vi "main.vi"() -> ()   [LabVIEW 2013]
uses:
  Controls/Soda Drinks.ctl
  Controls/Diet Soda Drinks.ctl
  Controls/Energy Drinks.ctl
  Controls/Alcohol Drinks.ctl
  Controls/Main UI Drinks.ctl
  Controls/Main Enum.ctl
panel:
  in  "cc?":bool
  out "CtlRef":refnum<vi>
  out "Label.Text":string
  in  "stop":bool
  in  "Reference Cluster":T1
  in  "UI":T2(tab)
  in  "All Selections":T3={"DaSani 20oz"=FALSE, "Mt. Dew 12oz"=FALSE, "Mt. Dew 20oz"=FALSE, "Diet Mt. Dew 20oz"=FALSE, "Pepsi 12oz"=FALSE, "Pepsi 20oz"=FALSE, "Diet Pepsi 20oz"=FALSE, "Sprite 12oz"=FALSE, "Sprite 20oz"=FALSE, "Dr. Pepper 12oz"=FALSE, "Dr. Pepper 20oz"=FALSE, "Lipton 16oz"=FALSE, "Starbucks 12oz"=FALSE, "Red Bull 8oz"=FALSE, "Coors 16oz"=FALSE, "Coors Light 16oz"=FALSE, "Hydra 12oz"=FALSE, "Diet Dr. Pepper 20oz"=FALSE, "Mt.Dew 12oz Price"=1.0, "Mt.Dew 20oz Price"=1.5, "Diet Mt.Dew 20oz Price"=1.5, "Pepsi 12oz Price"=1.0, "Pepsi 20oz Price"=1.5, "Diet Pepsi 20oz Price"=1.5, "Sprite 12oz Price"=1.0, "Sprite 20oz Price"=1.5, "Dr. Pepper 12oz Price"=1.0, "Dr. Pepper 20oz Price"=1.5, "Diet Dr. Pepper 20oz Price"=1.5, "DaSani 20oz Price"=1.0, "Lipton Prioce"=1.5, "Starbucks Price"=1.5, "Red Bull Price"=2.0, "Coors Price"=2.0, "Coors Light Price"=2.0, "Hydra Price"=2.0} {"Hydra Price" format="%.2g"; "Coors Light Price" format="%.2g"; "Coors Price" format="%.2g"; "Red Bull Price" format="%.2g"; "Starbucks Price" format="%.2g"; "Lipton Prioce" format="%.2g"; "DaSani 20oz Price" format="%.2g"; "Diet Dr. Pepper 20oz Price" format="%.2g"; "Dr. Pepper 20oz Price" format="%.2g"; "Dr. Pepper 12oz Price" format="%.2g"; "Sprite 20oz Price" format="%.2g"; "Sprite 12oz Price" format="%.2g"; "Diet Pepsi 20oz Price" format="%.2g"; "Pepsi 20oz Price" format="%.2g"; "Pepsi 12oz Price" format="%.2g"; "Diet Mt.Dew 20oz Price" format="%.2g"; "Mt.Dew 20oz Price" format="%.2g"; "Mt.Dew 12oz Price" format="%.2f"}
  in  "Energy":bool
  in  "Diet":bool
  in  "Alcohol":bool
  in  "Soda":bool
  in  "Add Money":bool
  out "Available Funds":dbl format="%.2f"
  in  "Return Money":bool
  out "Available Funds 2":dbl format="%.2f"
  in  "Imploded 1 Cancel":bool
  in  "Soda Drinks":T4={"DaSani 20oz"=FALSE, "Mt. Dew 12oz"=FALSE, "Mt. Dew 20oz"=FALSE, "Diet Mt. Dew 20oz"=FALSE, "Pepsi 12oz"=FALSE, "Pepsi 20oz"=FALSE, "Diet Pepsi 20oz"=FALSE, "Sprite 12oz"=FALSE, "Sprite 20oz"=FALSE, "Dr. Pepper 12oz"=FALSE, "Dr. Pepper 20oz"=FALSE, "Diet Dr. Pepper 20oz"=FALSE, "Mt.Dew 12oz Price"=1.0, "Mt.Dew 20oz Price"=1.5, "Diet Mt.Dew 20oz Price"=1.5, "Pepsi 12oz Price"=1.0, "Pepsi 20oz Price"=1.5, "Diet Pepsi 20oz Price"=1.5, "Sprite 12oz Price"=1.0, "Sprite 20oz Price"=1.5, "Dr. Pepper 12oz Price"=1.0, "Dr. Pepper 20oz Price"=1.5, "Diet Dr. Pepper 20oz Price"=1.5, "DaSani 20oz Price"=1.0} {"DaSani 20oz Price" format="%.2f"; "Diet Dr. Pepper 20oz Price" format="%.2f"; "Dr. Pepper 20oz Price" format="%.2f"; "Dr. Pepper 12oz Price" format="%.2f"; "Sprite 20oz Price" format="%.2f"; "Sprite 12oz Price" format="%.2f"; "Diet Pepsi 20oz Price" format="%.2f"; "Pepsi 20oz Price" format="%.2f"; "Pepsi 12oz Price" format="%.2f"; "Diet Mt.Dew 20oz Price" format="%.2f"; "Mt.Dew 20oz Price" format="%.2f"; "Mt.Dew 12oz Price" format="%.2f"}
  in  "Diet Selections":T5={"DaSani 20oz"=FALSE, "Diet Mt. Dew 20oz"=FALSE, "Diet Pepsi 20oz"=FALSE, "Diet Dr. Pepper 20oz"=FALSE, "Diet Mt.Dew 20oz Price"=1.5, "Diet Pepsi 20oz Price"=1.5, "Diet Dr. Pepper 20oz Price"=1.5, "DaSani 20oz Price"=1.0} {"DaSani 20oz Price" format="%.2f"; "Diet Dr. Pepper 20oz Price" format="%.2f"; "Diet Pepsi 20oz Price" format="%.2f"; "Diet Mt.Dew 20oz Price" format="%.2f"}
  in  "Energy Selections":T6={"Lipton 16oz"=FALSE, "Starbucks 12oz"=FALSE, "Red Bull 8oz"=FALSE, "Lipton Prioce"=1.5, "Starbucks Price"=1.5, "Red Bull Price"=2.0} {"Red Bull Price" format="%.2f"; "Starbucks Price" format="%.2f"; "Lipton Prioce" format="%.2f"}
  in  "Alcohol Drinks":T7={"Coors 16oz"=FALSE, "Coors Light 16oz"=FALSE, "Hydra 12oz"=FALSE, "Coors Price"=2.0, "Coors Light Price"=2.0, "Hydra Price"=2.0} {"Hydra Price" format="%.2f"; "Coors Light Price" format="%.2f"; "Coors Price" format="%.2f"}
  in  "Diet Implode":bool
  in  "Add Money 2":bool
  out "Available Funds 3":dbl format="%.2f"
  in  "Imploded 2 Cancel":bool
  in  "Diet Selections 2":T5={"DaSani 20oz"=FALSE, "Diet Mt. Dew 20oz"=FALSE, "Diet Pepsi 20oz"=FALSE, "Diet Dr. Pepper 20oz"=FALSE, "Diet Mt.Dew 20oz Price"=1.5, "Diet Pepsi 20oz Price"=1.5, "Diet Dr. Pepper 20oz Price"=1.5, "DaSani 20oz Price"=1.0} {"DaSani 20oz Price" format="%.2g"; "Diet Dr. Pepper 20oz Price" format="%.2g"; "Diet Pepsi 20oz Price" format="%.2g"; "Diet Mt.Dew 20oz Price" format="%.2g"}
  in  "Add Money 3":bool
  in  "Credit Card Cancel":bool
  in  "ID Scan Cancel":bool
  in  "Breath Cancel":bool
  in  "EXIT":bool
  # "In the actual implemented User Interface this lower section will not be developed.\nThis program is to only be used as a simulation of the application and how the UI \nshould work in various situations. \nAlso this is nowhere near a final UI it is a super duper rough draft :)\nMerely so I understand better what it is the system will accomplish."
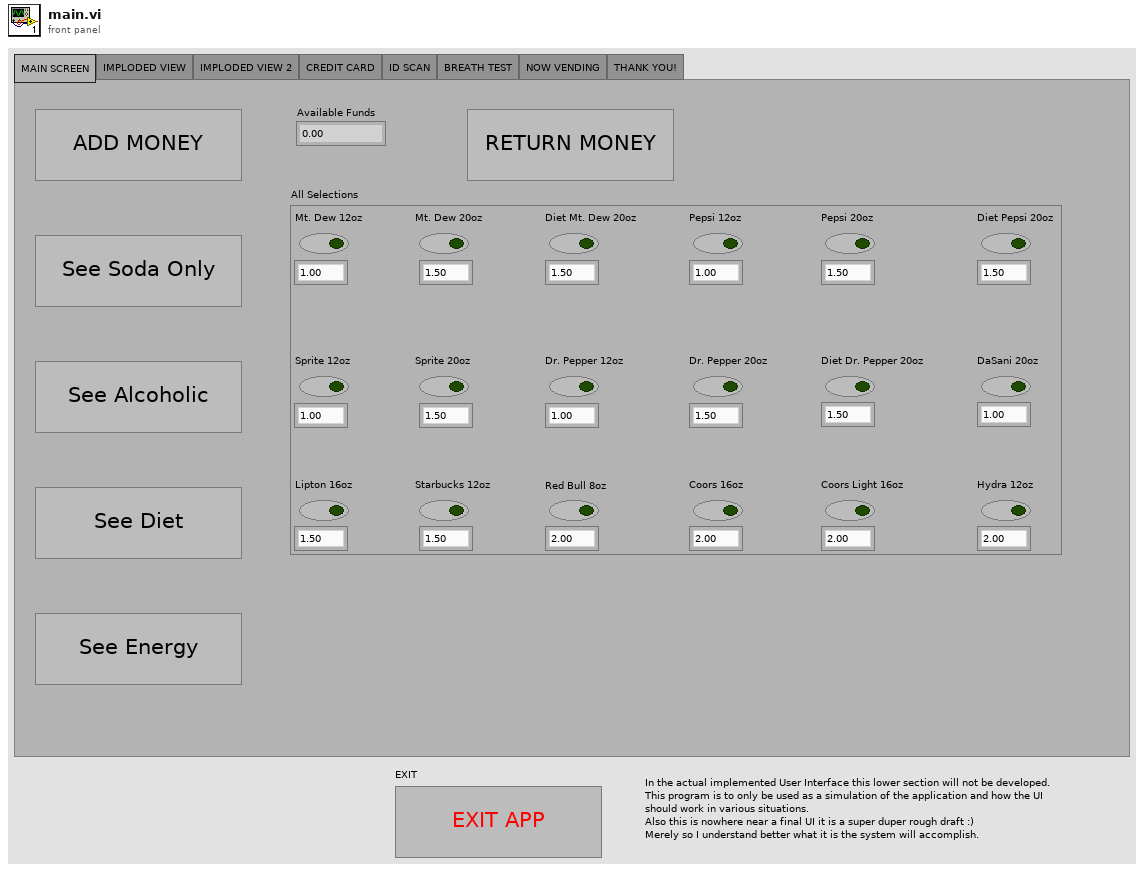
[diagram p1: front panel]
types:
  T1 = cluster{"Alcohol Drinks":refnum<vi>, "Energy Selections":refnum<vi>, "Diet Selections":refnum<vi>, "Soda Drinks":refnum<vi>}
  T2 = enum32{"MAIN SCREEN", "IMPLODED VIEW", "IMPLODED VIEW 2", "CREDIT CARD", "ID SCAN", "BREATH TEST", "NOW VENDING", "THANK YOU!"}
  T3 = typedef "Main UI Drinks.ctl" = cluster{"DaSani 20oz":bool, "Mt. Dew 12oz":bool, "Mt. Dew 20oz":bool, "Diet Mt. Dew 20oz":bool, "Pepsi 12oz":bool, "Pepsi 20oz":bool, "Diet Pepsi 20oz":bool, "Sprite 12oz":bool, "Sprite 20oz":bool, "Dr. Pepper 12oz":bool, "Dr. Pepper 20oz":bool, "Lipton 16oz":bool, "Starbucks 12oz":bool, "Red Bull 8oz":bool, "Coors 16oz":bool, "Coors Light 16oz":bool, "Hydra 12oz":bool, "Diet Dr. Pepper 20oz":bool, "Mt.Dew 12oz Price":dbl, "Mt.Dew 20oz Price":dbl, "Diet Mt.Dew 20oz Price":dbl, "Pepsi 12oz Price":dbl, "Pepsi 20oz Price":dbl, "Diet Pepsi 20oz Price":dbl, "Sprite 12oz Price":dbl, "Sprite 20oz Price":dbl, "Dr. Pepper 12oz Price":dbl, "Dr. Pepper 20oz Price":dbl, "Diet Dr. Pepper 20oz Price":dbl, "DaSani 20oz Price":dbl, "Lipton Prioce":dbl, "Starbucks Price":dbl, "Red Bull Price":dbl, "Coors Price":dbl, "Coors Light Price":dbl, "Hydra Price":dbl}
  T4 = typedef "Soda Drinks.ctl" = cluster{"DaSani 20oz":bool, "Mt. Dew 12oz":bool, "Mt. Dew 20oz":bool, "Diet Mt. Dew 20oz":bool, "Pepsi 12oz":bool, "Pepsi 20oz":bool, "Diet Pepsi 20oz":bool, "Sprite 12oz":bool, "Sprite 20oz":bool, "Dr. Pepper 12oz":bool, "Dr. Pepper 20oz":bool, "Diet Dr. Pepper 20oz":bool, "Mt.Dew 12oz Price":dbl, "Mt.Dew 20oz Price":dbl, "Diet Mt.Dew 20oz Price":dbl, "Pepsi 12oz Price":dbl, "Pepsi 20oz Price":dbl, "Diet Pepsi 20oz Price":dbl, "Sprite 12oz Price":dbl, "Sprite 20oz Price":dbl, "Dr. Pepper 12oz Price":dbl, "Dr. Pepper 20oz Price":dbl, "Diet Dr. Pepper 20oz Price":dbl, "DaSani 20oz Price":dbl}
  T5 = typedef "Diet Soda Drinks.ctl" = cluster{"DaSani 20oz":bool, "Diet Mt. Dew 20oz":bool, "Diet Pepsi 20oz":bool, "Diet Dr. Pepper 20oz":bool, "Diet Mt.Dew 20oz Price":dbl, "Diet Pepsi 20oz Price":dbl, "Diet Dr. Pepper 20oz Price":dbl, "DaSani 20oz Price":dbl}
  T6 = typedef "Energy Drinks.ctl" = cluster{"Lipton 16oz":bool, "Starbucks 12oz":bool, "Red Bull 8oz":bool, "Lipton Prioce":dbl, "Starbucks Price":dbl, "Red Bull Price":dbl}
  T7 = typedef "Alcohol Drinks.ctl" = cluster{"Coors 16oz":bool, "Coors Light 16oz":bool, "Hydra 12oz":bool, "Coors Price":dbl, "Coors Light Price":dbl, "Hydra Price":dbl}
  T8 = typedef "Main Enum.ctl" = enum8{"Initialize", "Timeout", "Add Money", "Return Money", "Implode Soda", "Implode Alcohol", "Implode Diet", "Implode Energy", "Secondary Implode", "Credit Card", "ID Scan", "Breath Test", "Vending", "Thanks!", "Reset to Default", "Exit", "Deinitialize"}
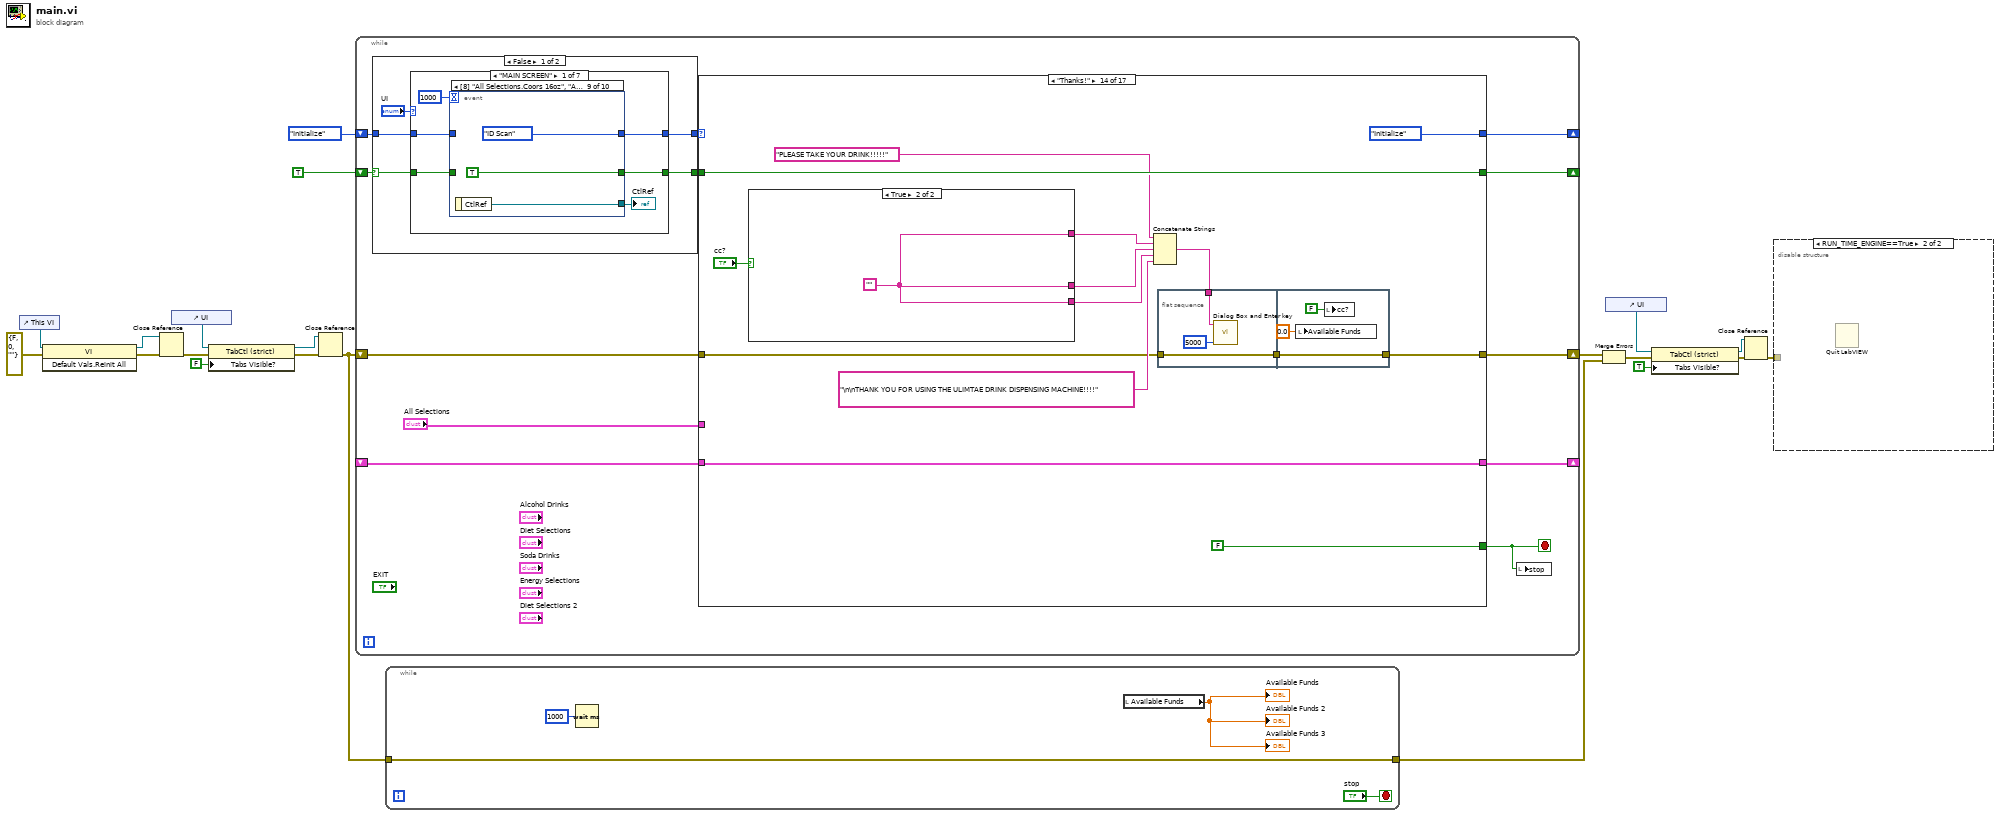
[diagram p0: block diagram]
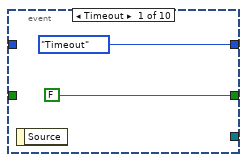
[diagram p3: hidden frame]
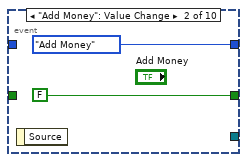
[diagram p4: hidden frame]
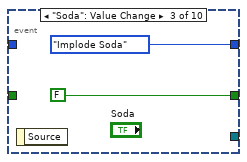
[diagram p5: hidden frame]
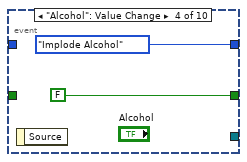
[diagram p6: hidden frame]
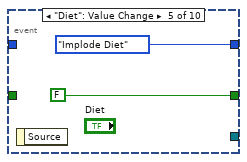
[diagram p7: hidden frame]
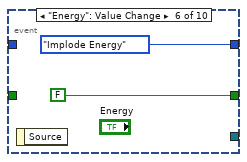
[diagram p8: hidden frame]
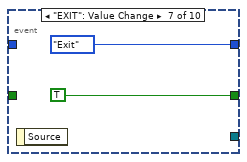
[diagram p9: hidden frame]
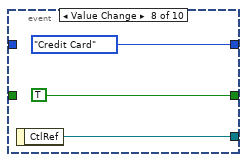
[diagram p10: hidden frame]
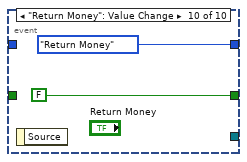
[diagram p11: hidden frame]
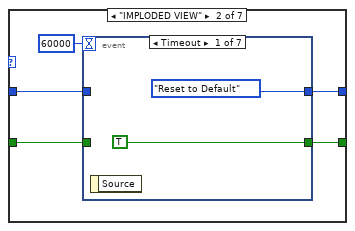
[diagram p12: hidden frame]
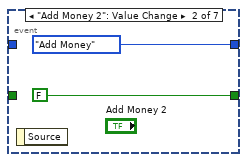
[diagram p13: hidden frame]
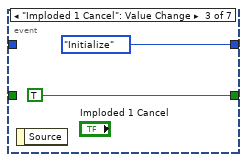
[diagram p14: hidden frame]
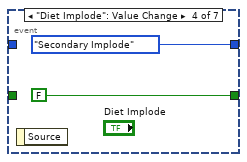
[diagram p15: hidden frame]
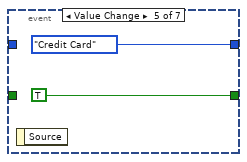
[diagram p16: hidden frame]
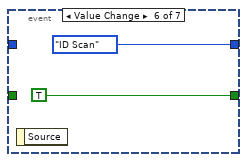
[diagram p17: hidden frame]
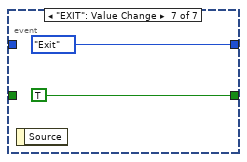
[diagram p18: hidden frame]
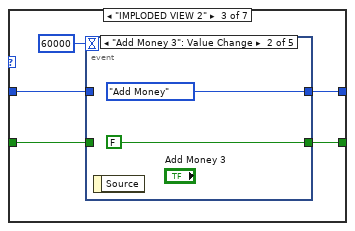
[diagram p19: hidden frame]
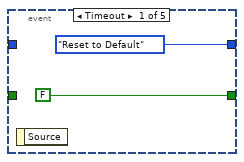
[diagram p20: hidden frame]
diagram:
  n1 = control-ref of="This VI"() -> (w3:refnum<vi>)
  n2 = invoke class="VI" method="Default Vals.Reinit All"(reference=w3, error in=errorcluster {"status"=FALSE, "code"=0, "source"=""} ("error constant")) -> (reference out=w5:refnum<vi>, error out=w4:errorcluster)  [unwired: 1 in, 1 out]
  n3 = Close Reference(reference=w5, error in (no error)=w4) -> (error out=w1:errorcluster)
  n4 = control-ref of="UI"() -> (w18:refnum<vi>)
  n5 = property class="TabCtl (strict)"(reference=w18, error in=w1, "Tabs Visible?"=FALSE) -> (reference out=w15:refnum<vi>, error out=w16:errorcluster)
  n6 = Close Reference(reference=w15, error in (no error)=w16) -> (error out=w7:errorcluster)
  n7 = while {
    shift-right: [w27] -> _
    shift-left: Main_Enum."Initialize" ("Enum") -> [w32]
    shift-right: [w28] -> _
    shift-left: TRUE -> [w31]
    shift-right: [w25] -> w9
    shift-left: w7 -> [w26]
    shift-right: [w22] -> _
    shift-left: _ -> [w23]
    stop <- w24 stop-if-true
    n8 = case shown="False" w31 {
      selector: w31 -> [w36 w135]
      tunnel: w32 -> [w35 w136]
      tunnel: [w34 w136] -> w29
      tunnel: [w33 w135] -> w30
      frame False {
        n9 = case shown="\"MAIN SCREEN\"" "UI" {
          tunnel: w36 -> [w41 w68 w87 w102 w113 w124 w133]
          tunnel: w35 -> [w42 w69 w88 w103 w114 w125 w134]
          tunnel: [w40 w67 w86 w101 w112 w123 w134] -> w34
          tunnel: [w39 w66 w85 w100 w111 w122 w133] -> w33
          frame "MAIN SCREEN" {
            n10 = event shown="[8] \"All Selections.Coors 16oz\", \"All Selections.Coors Light 16oz\", \"All Selections.Hydra 12oz\": Value Change" {
              selector: _ -> [_ _ _ _ _ _ _ _ _ _]
              dyn-events: _ -> [_ _ _ _ _ _ _ _ _ _]
              timeout: 1000 -> [_ _ _ _ _ _ _ _ _ _]
              tunnel: w42 -> [_ _ _ _ _ _ _ _ _ _]
              tunnel: w41 -> [_ _ _ _ _ _ _ _ _ _]
              tunnel: [Main_Enum."Timeout" ("Enum") Main_Enum."Add Money" ("Enum") Main_Enum."Implode Soda" ("Enum") Main_Enum."Implode Alcohol" ("Enum") Main_Enum."Implode Diet" ("Enum") Main_Enum."Implode Energy" ("Enum") Main_Enum."Exit" ("Enum") Main_Enum."Credit Card" ("Enum") Main_Enum."ID Scan" ("Enum") Main_Enum."Return Money" ("Enum")] -> w40
              tunnel: [FALSE FALSE FALSE FALSE FALSE FALSE TRUE TRUE TRUE FALSE] -> w39
              tunnel: [_ _ _ _ _ _ _ w58 w61 _] -> w38
              event Timeout {
                n11 = event-data() -> ()  [unwired: 1 in, 1 out]
              }
              event "Add Money": Value Change {
                n12 = event-data() -> ()  [unwired: 1 in, 1 out]
              }
              event "Soda": Value Change {
                n13 = event-data() -> ()  [unwired: 1 in, 1 out]
              }
              event "Alcohol": Value Change {
                n14 = event-data() -> ()  [unwired: 1 in, 1 out]
              }
              event "Diet": Value Change {
                n15 = event-data() -> ()  [unwired: 1 in, 1 out]
              }
              event "Energy": Value Change {
                n16 = event-data() -> ()  [unwired: 1 in, 1 out]
              }
              event "EXIT": Value Change {
                n17 = event-data() -> ()  [unwired: 1 in, 1 out]
              }
              event Value Change {
                n18 = event-data() -> ("CtlRef"=w58:refnum<vi>)  [unwired: 1 in]
              }
              event Value Change {
                n19 = event-data() -> ("CtlRef"=w61:refnum<vi>)  [unwired: 1 in]
              }
              event "Return Money": Value Change {
                n20 = event-data() -> ()  [unwired: 1 in, 1 out]
              }
            }
            "CtlRef" <- w38
          }
          frame "IMPLODED VIEW" {
            n21 = event shown="[0] Timeout" {
              selector: _ -> [_ _ _ _ _ _ _]
              dyn-events: _ -> [_ _ _ _ _ _ _]
              timeout: 60000 -> [_ _ _ _ _ _ _]
              tunnel: w69 -> [_ _ _ _ _ _ _]
              tunnel: w68 -> [_ _ _ _ _ _ _]
              tunnel: [Main_Enum."Reset to Default" ("Enum") Main_Enum."Add Money" ("Enum") Main_Enum."Initialize" ("Enum") Main_Enum."Secondary Implode" ("Enum") Main_Enum."Credit Card" ("Enum") Main_Enum."ID Scan" ("Enum") Main_Enum."Exit" ("Enum")] -> w67
              tunnel: [TRUE FALSE TRUE FALSE TRUE TRUE TRUE] -> w66
              event Timeout {
                n22 = event-data() -> ()  [unwired: 1 in, 1 out]
              }
              event "Add Money 2": Value Change {
                n23 = event-data() -> ()  [unwired: 1 in, 1 out]
              }
              event "Imploded 1 Cancel": Value Change {
                n24 = event-data() -> ()  [unwired: 1 in, 1 out]
              }
              event "Diet Implode": Value Change {
                n25 = event-data() -> ()  [unwired: 1 in, 1 out]
              }
              event Value Change {
                n26 = event-data() -> ()  [unwired: 1 in, 1 out]
              }
              event Value Change {
                n27 = event-data() -> ()  [unwired: 1 in, 1 out]
              }
              event "EXIT": Value Change {
                n28 = event-data() -> ()  [unwired: 1 in, 1 out]
              }
            }
          }
          frame "IMPLODED VIEW 2" {
            n29 = event shown="[1] \"Add Money 3\": Value Change" {
              selector: _ -> [_ _ _ _ _]
              dyn-events: _ -> [_ _ _ _ _]
              timeout: 60000 -> [_ _ _ _ _]
              tunnel: w88 -> [_ _ _ _ _]
              tunnel: w87 -> [_ _ _ _ _]
              tunnel: [Main_Enum."Reset to Default" ("Enum") Main_Enum."Add Money" ("Enum") Main_Enum."Implode Soda" ("Enum") Main_Enum."Exit" ("Enum") Main_Enum."Credit Card" ("Enum")] -> w86
              tunnel: [FALSE FALSE FALSE TRUE TRUE] -> w85
              event Timeout {
                n30 = event-data() -> ()  [unwired: 1 in, 1 out]
              }
              event "Add Money 3": Value Change {
                n31 = event-data() -> ()  [unwired: 1 in, 1 out]
              }
              event "Imploded 2 Cancel": Value Change {
                n32 = event-data() -> ()  [unwired: 1 in, 1 out]
              }
              event "EXIT": Value Change {
                n33 = event-data() -> ()  [unwired: 1 in, 1 out]
              }
              event Value Change {
                n34 = event-data() -> ()  [unwired: 1 in, 1 out]
              }
            }
          }
          frame "CREDIT CARD" {
            n35 = event shown="[2] \"EXIT\": Value Change" {
              selector: _ -> [_ _ _]
              dyn-events: _ -> [_ _ _]
              timeout: 60000 -> [_ _ _]
              tunnel: w103 -> [_ _ _]
              tunnel: w102 -> [_ _ _]
              tunnel: [Main_Enum."Reset to Default" ("Enum") Main_Enum."Timeout" ("Enum") Main_Enum."Exit" ("Enum")] -> w101
              tunnel: [FALSE FALSE TRUE] -> w100
              event Timeout {
                n36 = event-data() -> ()  [unwired: 1 in, 1 out]
              }
              event "Credit Card Cancel": Value Change {
                n37 = event-data() -> ()  [unwired: 1 in, 1 out]
              }
              event "EXIT": Value Change {
                n38 = event-data() -> ()  [unwired: 1 in, 1 out]
              }
            }
          }
          frame "ID SCAN" {
            n39 = event shown="[0] Timeout" {
              selector: _ -> [_ _ _]
              dyn-events: _ -> [_ _ _]
              timeout: 60000 -> [_ _ _]
              tunnel: w114 -> [_ _ _]
              tunnel: w113 -> [_ _ _]
              tunnel: [Main_Enum."Reset to Default" ("Enum") Main_Enum."Timeout" ("Enum") Main_Enum."Exit" ("Enum")] -> w112
              tunnel: [FALSE FALSE TRUE] -> w111
              event Timeout {
                n40 = event-data() -> ()  [unwired: 1 in, 1 out]
              }
              event "ID Scan Cancel": Value Change {
                n41 = event-data() -> ()  [unwired: 1 in, 1 out]
              }
              event "EXIT": Value Change {
                n42 = event-data() -> ()  [unwired: 1 in, 1 out]
              }
            }
          }
          frame "BREATH TEST" {
            n43 = event shown="[0] Timeout" {
              selector: _ -> [_ _ _]
              dyn-events: _ -> [_ _ _]
              timeout: 60000 -> [_ _ _]
              tunnel: w125 -> [_ _ _]
              tunnel: w124 -> [_ _ _]
              tunnel: [Main_Enum."Reset to Default" ("Enum") Main_Enum."Timeout" ("Enum") Main_Enum."Exit" ("Enum")] -> w123
              tunnel: [FALSE FALSE TRUE] -> w122
              event Timeout {
                n44 = event-data() -> ()  [unwired: 1 in, 1 out]
              }
              event "Breath Cancel": Value Change {
                n45 = event-data() -> ()  [unwired: 1 in, 1 out]
              }
              event "EXIT": Value Change {
                n46 = event-data() -> ()  [unwired: 1 in, 1 out]
              }
            }
          }
          frame "NOW VENDING", Default {
          }
        }
      }
      frame True {
      }
    }
    n47 = case shown="\"Thanks!\"" w29 {
      selector: w29 -> [_ w180 _ w202 w218 w244 w270 w296 w319 _ _ _ w445 _ _ w494 w496]
      tunnel: w30 -> [w152 _ w190 w201 w217 w243 w269 w295 w318 w334 w419 w435 w449 w463 w485 w490 w503]
      tunnel: [w152 FALSE w190 w201 w217 w243 w269 w295 w318 w334 w419 w435 w449 w463 w485 w490 w503] -> w28
      tunnel: [Main_Enum."Timeout" w180 Main_Enum."Timeout" ("Enum") w202 w218 w244 w270 w296 w319 w330 w416 w431 w444 Main_Enum."Initialize" ("Enum") Main_Enum."Initialize" ("Enum") w493 w496] -> w27
      tunnel: w26 -> [w137 w179 w189 w203 w213 w239 w266 w292 w317 w333 w412 w430 w448 w456 w488 w491 w501]
      tunnel: [w143 w179 w185 w197 w206 w238 w263 w290 w317 w328 w415 w432 w448 w455 w488 w491 w497] -> w25
      tunnel: [w138 w176 w182 w200 w212 w237 w265 w289 w316 w336 w418 w434 w447 w462 w487 w492 T1 {"Alcohol Drinks"=refnum, "Energy Selections"=refnum, "Diet Selections"=refnum, "Soda Drinks"=refnum} ("Reference Cluster")] -> w22
      tunnel: w23 -> [_ w176 w182 w200 w212 w237 w265 w289 w316 w336 w418 w434 w447 w462 w487 w492 _]
      tunnel: [FALSE FALSE FALSE FALSE FALSE FALSE FALSE FALSE FALSE FALSE FALSE FALSE FALSE FALSE FALSE FALSE TRUE] -> w24
      tunnel: "All Selections" -> [_ _ _ _ _ _ _ _ _ w323 _ _ _ _ _ _ _]
      frame "Initialize", Default {
        n48 = control-ref of="Alcohol Drinks"() -> (w142:refnum<vi>)
        n49 = control-ref of="Energy Selections"() -> (w141:refnum<vi>)
        n50 = control-ref of="Diet Selections"() -> (w140:refnum<vi>)
        n51 = control-ref of="Soda Drinks"() -> (w139:refnum<vi>)
        n52 = Bundle By Name(cluster="Reference Cluster", "Alcohol Drinks"=w142, "Energy Selections"=w141, "Diet Selections"=w140, "Soda Drinks"=w139) -> (w138:T1)
        n53 = for {
          N: 4 -> [_]
          tunnel: w137 -> [w163]
          tunnel: w138 -> [w161]
          tunnel: [w155] -> w144
          i -> [w162]
          n54 = case shown="0, Default" w162 {
            tunnel: w163 -> [w165 w168 w171 w174]
            tunnel: w161 -> [w166 w169 w172 w175]
            tunnel: [w165 w168 w171 w174] -> w160
            tunnel: [w164 w167 w170 w173] -> w159
            frame 0, Default {
              n55 = Unbundle By Name(w166) -> ("Soda Drinks"=w164:refnum<vi>)
            }
            frame 1 {
              n56 = Unbundle By Name(w169) -> ("Alcohol Drinks"=w167:refnum<vi>)
            }
            frame 2 {
              n57 = Unbundle By Name(w172) -> ("Diet Selections"=w170:refnum<vi>)
            }
            frame 3 {
              n58 = Unbundle By Name(w175) -> ("Energy Selections"=w173:refnum<vi>)
            }
          }
          n59 = property class="Clust"(reference=w159, error in=w160, "Visible"=TRUE) -> (reference out=w156:refnum<vi>, error out=w157:errorcluster)
          n60 = Close Reference(reference=w156, error in (no error)=w157) -> (error out=w155:errorcluster)
        }
        n61 = local write "UI"(T2."MAIN SCREEN" ("UI")) -> ()
        n62 = control-ref of="Diet Implode"() -> (w145:refnum<vi>)
        n63 = property class="Bool"(reference=w145, error in=w144, "Visible"=FALSE) -> (reference out=w148:refnum<vi>, error out=w147:errorcluster)
        n64 = Close Reference(reference=w148, error in (no error)=w147) -> (error out=w143:errorcluster)
      }
      frame "Timeout" {
        n65 = local write "UI"(T2."MAIN SCREEN" ("UI")) -> ()
      }
      frame "Add Money" {
        # "Need Global Here"
        n66 = call "Prompt User for Input"("error in (no error)"=w189) -> ("Money"=w187:dbl, "error out"=w185:errorcluster)  [unwired: 16 in, 1 out]
        n67 = local read "Available Funds"() -> (w188:dbl)
        n68 = Add(x=w188, y=w187) -> (x+y=w186:dbl)
        n69 = local write "Available Funds"(w186) -> ()
      }
      frame "Return Money" {
        n70 = local read "Available Funds"() -> (w193:dbl)
        n71 = Number To Fractional String(number=w193, precision (6)=i16 2) -> (F-format string=w192:string)  [unwired: 2 in]
        n72 = Concatenate Strings("Please take your money from the return coin slot.\n\nThere is $" ("Message"), w192, " in the return coin slot." ("Message")) -> (w194:string)
        n73 = call "Display Message to User"("error in (no error)"=w203, "Message"=w194) -> ("error out"=w198:errorcluster)  [unwired: 8 in, 1 out]
        n74 = flat-sequence {
          tunnel: w198 -> [w204]
          tunnel: [w204] -> w197
          frame #0 {
            n75 = local write "Available Funds"(0.0 ("Available Funds")) -> ()
          }
        }
      }
      frame "Implode Soda" {
        n76 = for {
          N: 3 -> [_]
          tunnel: w213 -> [w227]
          tunnel: w212 -> [w225]
          tunnel: [w219] -> w207
          i -> [w226]
          n77 = case shown="0, Default" w226 {
            tunnel: w227 -> [w229 w232 w235]
            tunnel: w225 -> [w230 w233 w236]
            tunnel: [w229 w232 w235] -> w224
            tunnel: [w228 w231 w234] -> w223
            frame 0, Default {
              n78 = Unbundle By Name(w230) -> ("Alcohol Drinks"=w228:refnum<vi>)
            }
            frame 1 {
              n79 = Unbundle By Name(w233) -> ("Diet Selections"=w231:refnum<vi>)
            }
            frame 2 {
              n80 = Unbundle By Name(w236) -> ("Energy Selections"=w234:refnum<vi>)
            }
          }
          n81 = property class="Clust"(reference=w223, error in=w224, "Visible"=FALSE) -> (reference out=w220:refnum<vi>, error out=w221:errorcluster)
          n82 = Close Reference(reference=w220, error in (no error)=w221) -> (error out=w219:errorcluster)
        }
        n83 = local write "UI"(T2."IMPLODED VIEW" ("UI")) -> ()
        n84 = control-ref of="Diet Implode"() -> (w208:refnum<vi>)
        n85 = property class="Bool"(reference=w208, error in=w207, "Visible"=TRUE) -> (reference out=w211:refnum<vi>, error out=w210:errorcluster)
        n86 = Close Reference(reference=w211, error in (no error)=w210) -> (error out=w206:errorcluster)
      }
      frame "Implode Alcohol" {
        n87 = for {
          N: 3 -> [_]
          tunnel: w239 -> [w253]
          tunnel: w237 -> [w251]
          tunnel: [w245] -> w238
          i -> [w252]
          n88 = case shown="2" w252 {
            tunnel: w253 -> [w255 w258 w261]
            tunnel: w251 -> [w256 w259 w262]
            tunnel: [w255 w258 w261] -> w250
            tunnel: [w254 w257 w260] -> w249
            frame 0, Default {
              n89 = Unbundle By Name(w256) -> ("Soda Drinks"=w254:refnum<vi>)
            }
            frame 1 {
              n90 = Unbundle By Name(w259) -> ("Diet Selections"=w257:refnum<vi>)
            }
            frame 2 {
              n91 = Unbundle By Name(w262) -> ("Energy Selections"=w260:refnum<vi>)
            }
          }
          n92 = property class="Clust"(reference=w249, error in=w250, "Visible"=FALSE) -> (reference out=w246:refnum<vi>, error out=w247:errorcluster)
          n93 = Close Reference(reference=w246, error in (no error)=w247) -> (error out=w245:errorcluster)
        }
        n94 = local write "UI"(T2."IMPLODED VIEW" ("UI")) -> ()
      }
      frame "Implode Diet" {
        n95 = for {
          N: 3 -> [_]
          tunnel: w266 -> [w279]
          tunnel: w265 -> [w277]
          tunnel: [w271] -> w263
          i -> [w278]
          n96 = case shown="2" w278 {
            tunnel: w279 -> [w281 w284 w287]
            tunnel: w277 -> [w282 w285 w288]
            tunnel: [w281 w284 w287] -> w276
            tunnel: [w280 w283 w286] -> w275
            frame 0, Default {
              n97 = Unbundle By Name(w282) -> ("Soda Drinks"=w280:refnum<vi>)
            }
            frame 1 {
              n98 = Unbundle By Name(w285) -> ("Alcohol Drinks"=w283:refnum<vi>)
            }
            frame 2 {
              n99 = Unbundle By Name(w288) -> ("Energy Selections"=w286:refnum<vi>)
            }
          }
          n100 = property class="Clust"(reference=w275, error in=w276, "Visible"=FALSE) -> (reference out=w272:refnum<vi>, error out=w273:errorcluster)
          n101 = Close Reference(reference=w272, error in (no error)=w273) -> (error out=w271:errorcluster)
        }
        n102 = local write "UI"(T2."IMPLODED VIEW" ("UI")) -> ()
      }
      frame "Implode Energy" {
        n103 = for {
          N: 3 -> [_]
          tunnel: w292 -> [w305]
          tunnel: w289 -> [w303]
          tunnel: [w297] -> w290
          i -> [w304]
          n104 = case shown="0, Default" w304 {
            tunnel: w305 -> [w307 w310 w313]
            tunnel: w303 -> [w308 w311 w314]
            tunnel: [w307 w310 w313] -> w302
            tunnel: [w306 w309 w312] -> w301
            frame 0, Default {
              n105 = Unbundle By Name(w308) -> ("Soda Drinks"=w306:refnum<vi>)
            }
            frame 1 {
              n106 = Unbundle By Name(w311) -> ("Alcohol Drinks"=w309:refnum<vi>)
            }
            frame 2 {
              n107 = Unbundle By Name(w314) -> ("Diet Selections"=w312:refnum<vi>)
            }
          }
          n108 = property class="Clust"(reference=w301, error in=w302, "Visible"=FALSE) -> (reference out=w298:refnum<vi>, error out=w299:errorcluster)
          n109 = Close Reference(reference=w298, error in (no error)=w299) -> (error out=w297:errorcluster)
        }
        n110 = local write "UI"(T2."IMPLODED VIEW" ("UI")) -> ()
      }
      frame "Secondary Implode" {
        n111 = local write "UI"(T2."IMPLODED VIEW 2" ("UI")) -> ()
      }
      frame "Credit Card" {
        # "Need to figure out how to delete price and if 0 use a credit card"
        n112 = local read "CtlRef"() -> (w327:refnum<vi>)
        n113 = local read "Available Funds"() -> (w321:dbl)
        n114 = property class="Ctl"(reference=w327, error in=w333) -> (reference out=w331:refnum<vi>, error out=w332:errorcluster, "Label.Text"=w324:string)
        "Label.Text" <- w324
        n115 = Close Reference(reference=w331, error in (no error)=w332) -> (error out=w329:errorcluster)
        n116 = case shown="\"Hydra 12oz\"" w324 {
          tunnel: w323 -> [_ w339 w341 w343 w345 w347 w349 w351 w353 w355 w357 w359 w361 w363 w365 w367 w369 w371 w373]
          tunnel: [0.0 ("Mt.Dew 12oz Price") w338 w340 w342 w344 w346 w348 w350 w352 w354 w356 w358 w360 w362 w364 w366 w368 w370 w372] -> w322
          frame "False", Default {
          }
          frame "Mt. Dew 12oz" {
            n117 = Unbundle By Name(w339) -> ("Mt.Dew 12oz Price"=w338:dbl)
          }
          frame "Mt. Dew 20oz" {
            n118 = Unbundle By Name(w341) -> ("Mt.Dew 20oz Price"=w340:dbl)
          }
          frame "Diet Mt. Dew 20oz" {
            n119 = Unbundle By Name(w343) -> ("Diet Mt.Dew 20oz Price"=w342:dbl)
          }
          frame "Pepsi 12oz" {
            n120 = Unbundle By Name(w345) -> ("Pepsi 12oz Price"=w344:dbl)
          }
          frame "Pepsi 20oz" {
            n121 = Unbundle By Name(w347) -> ("Pepsi 20oz Price"=w346:dbl)
          }
          frame "Diet Pepsi 20oz" {
            n122 = Unbundle By Name(w349) -> ("Diet Pepsi 20oz Price"=w348:dbl)
          }
          frame "Sprite 12oz" {
            n123 = Unbundle By Name(w351) -> ("Sprite 12oz Price"=w350:dbl)
          }
          frame "Sprite 20oz" {
            n124 = Unbundle By Name(w353) -> ("Sprite 20oz Price"=w352:dbl)
          }
          frame "Dr. Pepper 12oz" {
            n125 = Unbundle By Name(w355) -> ("Dr. Pepper 12oz Price"=w354:dbl)
          }
          frame "Dr. Pepper 20oz" {
            n126 = Unbundle By Name(w357) -> ("Dr. Pepper 20oz Price"=w356:dbl)
          }
          frame "Diet Dr. Pepper 20oz" {
            n127 = Unbundle By Name(w359) -> ("Diet Dr. Pepper 20oz Price"=w358:dbl)
          }
          frame "DaSani 20oz" {
            n128 = Unbundle By Name(w361) -> ("DaSani 20oz Price"=w360:dbl)
          }
          frame "Lipton 16oz" {
            n129 = Unbundle By Name(w363) -> ("Lipton Prioce"=w362:dbl)
          }
          frame "Starbucks 12oz" {
            n130 = Unbundle By Name(w365) -> ("Starbucks Price"=w364:dbl)
          }
          frame "Red Bull 8oz" {
            n131 = Unbundle By Name(w367) -> ("Red Bull Price"=w366:dbl)
          }
          frame "Coors 16oz" {
            n132 = Unbundle By Name(w369) -> ("Coors Price"=w368:dbl)
          }
          frame "Coors Light 16oz" {
            n133 = Unbundle By Name(w371) -> ("Coors Light Price"=w370:dbl)
          }
          frame "Hydra 12oz" {
            n134 = Unbundle By Name(w373) -> ("Hydra Price"=w372:dbl)
          }
        }
        n135 = Equal?(x=w321, y=0.0) -> (x = y?=w325:bool)
        n136 = local write "cc?"(w325) -> ()
        n137 = case shown="False" w325 {
          tunnel: [w376 w399] -> w330
          tunnel: w329 -> [w379 w397]
          tunnel: [w377 w398] -> w328
          tunnel: w322 -> [w380 w394]
          tunnel: w321 -> [w374 _]
          frame False {
            n138 = Subtract(x=w374, y=w380) -> (x-y=w375:dbl)
            n139 = local write "Available Funds"(w375) -> ()
            n140 = Greater Or Equal To 0?(x=w375) -> (x >= 0?=w378:bool)
            n141 = case shown="True" w378 {
              tunnel: w379 -> [w389 w393]
              tunnel: [w389 w393] -> w377
              tunnel: [Main_Enum."Initialize" ("Enum") Main_Enum."Vending" ("Enum")] -> w376
              tunnel: w375 -> [w388 _]
              tunnel: w374 -> [w381 _]
              frame False {
                n142 = Negate(x=w388) -> (-x=w384:dbl)
                n143 = local write "Available Funds"(w381) -> ()
                n144 = Number To Fractional String(number=w384, precision (6)=i16 2) -> (F-format string=w383:string)  [unwired: 2 in]
                n145 = Concatenate Strings("You are short by $" ("message"), w383, "\n\nPlease insert more money! " ("message")) -> (w387:string)
                n146 = call "Dialog Box and Enter key.vi"("milliseconds to wait"=u32 2000, "message"=w387) -> ()  [unwired: 10 in]
              }
              frame True {
              }
            }
          }
          frame True {
            n147 = call "Display Message to User2"("error in (no error)"=w397) -> ("error out"=w395:errorcluster, "Valid"=w396:bool)  [unwired: 9 in]
            n148 = case shown="False" w396 {
              tunnel: [Main_Enum."Initialize" ("Enum") Main_Enum."Vending" ("Enum")] -> w399
              tunnel: w395 -> [w400 w409]
              tunnel: [w400 w409] -> w398
              tunnel: w394 -> [_ w404]
              frame False {
                n149 = call "Dialog Box and Enter key.vi"("milliseconds to wait"=u32 2000, "message"="INVALID FUNDS ON CREDIT CARD!!!") -> ()  [unwired: 10 in]
              }
              frame True {
                n150 = Number To Fractional String(number=w404, precision (6)=i16 2) -> (F-format string=w405:string)  [unwired: 2 in]
                n151 = Concatenate Strings("Your card hase been charged $" ("message"), w405) -> (w407:string)
                n152 = call "Dialog Box and Enter key.vi"("milliseconds to wait"=u32 2000, "message"=w407) -> ()  [unwired: 10 in]
              }
            }
          }
        }
      }
      frame "ID Scan" {
        n153 = call "Display Message to User3"("error in (no error)"=w412) -> ("error out"=w414:errorcluster, "PASS"=w413:bool)  [unwired: 9 in]
        n154 = case shown="True" w413 {
          tunnel: [Main_Enum."Initialize" ("Enum") Main_Enum."Breath Test" ("Enum")] -> w416
          tunnel: w414 -> [w420 w424]
          tunnel: [w420 w424] -> w415
          frame False {
            n155 = call "Dialog Box and Enter key.vi"("milliseconds to wait"=u32 2000, "message"="ID SCAN FAILS!!!! RESTTING SYSTEM!!") -> ()  [unwired: 10 in]
          }
          frame True {
          }
        }
      }
      frame "Breath Test" {
        n156 = call "BAC ENTRY2"("error in (no error)"=w430) -> ("BAC"=w429:dbl, "error out"=w426:errorcluster)  [unwired: 16 in, 1 out]
        n157 = Less Or Equal?(x=w429, y=0.08) -> (x <= y?=w428:bool)
        n158 = case shown="False" w428 {
          tunnel: w426 -> [w436 w441]
          tunnel: [w436 w441] -> w432
          tunnel: [Main_Enum."Initialize" ("Enum") Main_Enum."Credit Card" ("Enum")] -> w431
          frame False {
            n159 = call "Dialog Box and Enter key.vi"("milliseconds to wait"=u32 2000, "message"="SORRY YOU ARE DRUNK!!!\n\nNO DRINK FOR YOU!") -> ()  [unwired: 10 in]
          }
          frame True {
          }
        }
      }
      frame "Vending" {
        n160 = Increment(x=w445) -> (x+1=w444:T8)
        n161 = call "Dialog Box and Enter key.vi"("milliseconds to wait"=u32 2000, "message"="NOW VENDING YOUR DRINK") -> ()  [unwired: 10 in]
      }
      frame "Thanks!" {
        n162 = case shown="True" "cc?" {
          tunnel: [w468 w475] -> w459
          tunnel: [w467 w475] -> w458
          tunnel: [w466 w475] -> w450
          frame False {
            n163 = local read "Available Funds"() -> (w465:dbl)
            n164 = Greater Than 0?(x=w465) -> (x > 0?=w464:bool)
            n165 = case shown="True" w464 {
              tunnel: [w469 w473] -> w468
              tunnel: [w469 " in the return coin slot." ("Message")] -> w467
              tunnel: [w469 "Please take the $" ("message")] -> w466
              tunnel: w465 -> [_ w470]
              frame False {
                w469 = ""
              }
              frame True {
                n166 = Number To Fractional String(number=w470, precision (6)=i16 2) -> (F-format string=w473:string)  [unwired: 2 in]
              }
            }
          }
          frame True {
            w475 = ""
          }
        }
        n167 = Concatenate Strings("PLEASE TAKE YOUR DRINK!!!!!" ("message"), w450, w459, w458, "\n\nTHANK YOU FOR USING THE ULIMTAE DRINK DISPENSING MACHINE!!!!" ("message")) -> (w453:string)
        n168 = flat-sequence {
          tunnel: w456 -> [w478]
          tunnel: [w478] -> w454
          tunnel: w453 -> [w476]
          tunnel: [w480] -> w455
          tunnel: w454 -> [w480]
          frame #0 {
            n169 = call "Dialog Box and Enter key.vi"("milliseconds to wait"=u32 5000, "message"=w476) -> ()  [unwired: 10 in]
          }
          frame #1 {
            n170 = local write "Available Funds"(0.0 ("Available Funds")) -> ()
            n171 = local write "cc?"(FALSE ("cc?")) -> ()
          }
        }
      }
      frame "Reset to Default" {
        n172 = call "Dialog Box and Enter key.vi"("milliseconds to wait"=u32 5000, "message"="SYSTEM TIMEOUT OCCURED. NOW RESETTING TO DEFAULT SETTINGS.\nYORU MONEY AMOUNT WILL BE MAINTAINED") -> ()  [unwired: 10 in]
      }
      frame "Exit" {
        n173 = Increment(x=w494) -> (x+1=w493:T8)
      }
      frame "Deinitialize" {
        n174 = control-ref of="This VI"() -> (w500:refnum<vi>)
        n175 = invoke class="VI" method="Default Vals.Reinit All"(reference=w500, error in=w501) -> (reference out=w498:refnum<vi>, error out=w499:errorcluster)  [unwired: 1 in, 1 out]
        n176 = Close Reference(reference=w498, error in (no error)=w499) -> (error out=w497:errorcluster)
      }
    }
    n177 = local write "stop"(w24) -> ()
  }
  n178 = while {
    tunnel: w7 -> [w504]
    tunnel: [w504] -> w6
    stop <- "stop" stop-if-true
    n179 = Wait (ms)(milliseconds to wait=u32 1000) -> ()  [unwired: 1 out]
    n180 = local read "Available Funds"() -> (→"Available Funds" →"Available Funds 3" →"Available Funds 2":dbl)
  }
  n181 = Merge Errors(w9, w6) -> (w8:errorcluster)
  n182 = control-ref of="UI"() -> (w11:refnum<vi>)
  n183 = property class="TabCtl (strict)"(reference=w11, error in=w8, "Tabs Visible?"=TRUE) -> (reference out=w14:refnum<vi>, error out=w13:errorcluster)
  n184 = Close Reference(reference=w14, error in (no error)=w13) -> (error out=w10:errorcluster)
  n185 = disable-structure shown="RUN_TIME_ENGINE==True" {
    disable-tunnel: w10 -> [_ _]
    frame condition #0 (active) {
    }
    frame condition #1 {
      n186 = Quit LabVIEW() -> ()  [unwired: 1 in]
    }
  }
